vi "Scan Engine EtherCAT Slave.vi"(8 "error in (no error)":errorcluster, 11 "Node Ptr":T1 format="%.0x") -> (0 "error out":errorcluster)   [LabVIEW 2020, in "SEECD System Explorer.lvlib"]
uses:
  SEECD System Explorer.lvlib
  <vilib>/NI VeriStand/Custom Device API/Custom Device API.lvlib
  Shared/Globals/Property Strings.vi
  Shared/SEECD Shared.lvlib
  <vilib>/NI VeriStand/Custom Device API/Set Item Property (U16).vi
  <vilib>/NI VeriStand/Custom Device API/Set Item Property (Boolean).vi
  <vilib>/NI VeriStand/Custom Device API/Custom Device Item Ref.ctl
panel:
  in  "Prepend":bool caption="Prepend slave position to name"
  in  "SHDocVw.IWebBrowser2":refnum<k7>(container)
  in  "Slave Position":u16
  in  "Header":cluster{"Section Name":string}={"Section Name"="NI-914x Chassis"}
  in  "Name":string
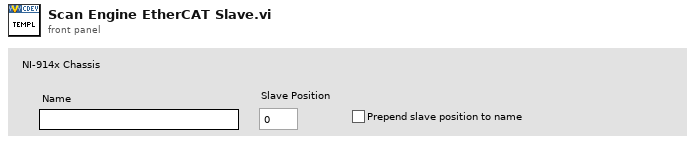
[diagram p1: front panel]
types:
  T1 = typedef "Custom Device API.lvlib/Custom Device Item Ref.ctl" = u64
  T2 = typedef "Custom Device API.lvlib/Custom Device Commands.ctl" = enum16{"Default", "Item renamed", "Shutdown", "Dynamic button pressed"}
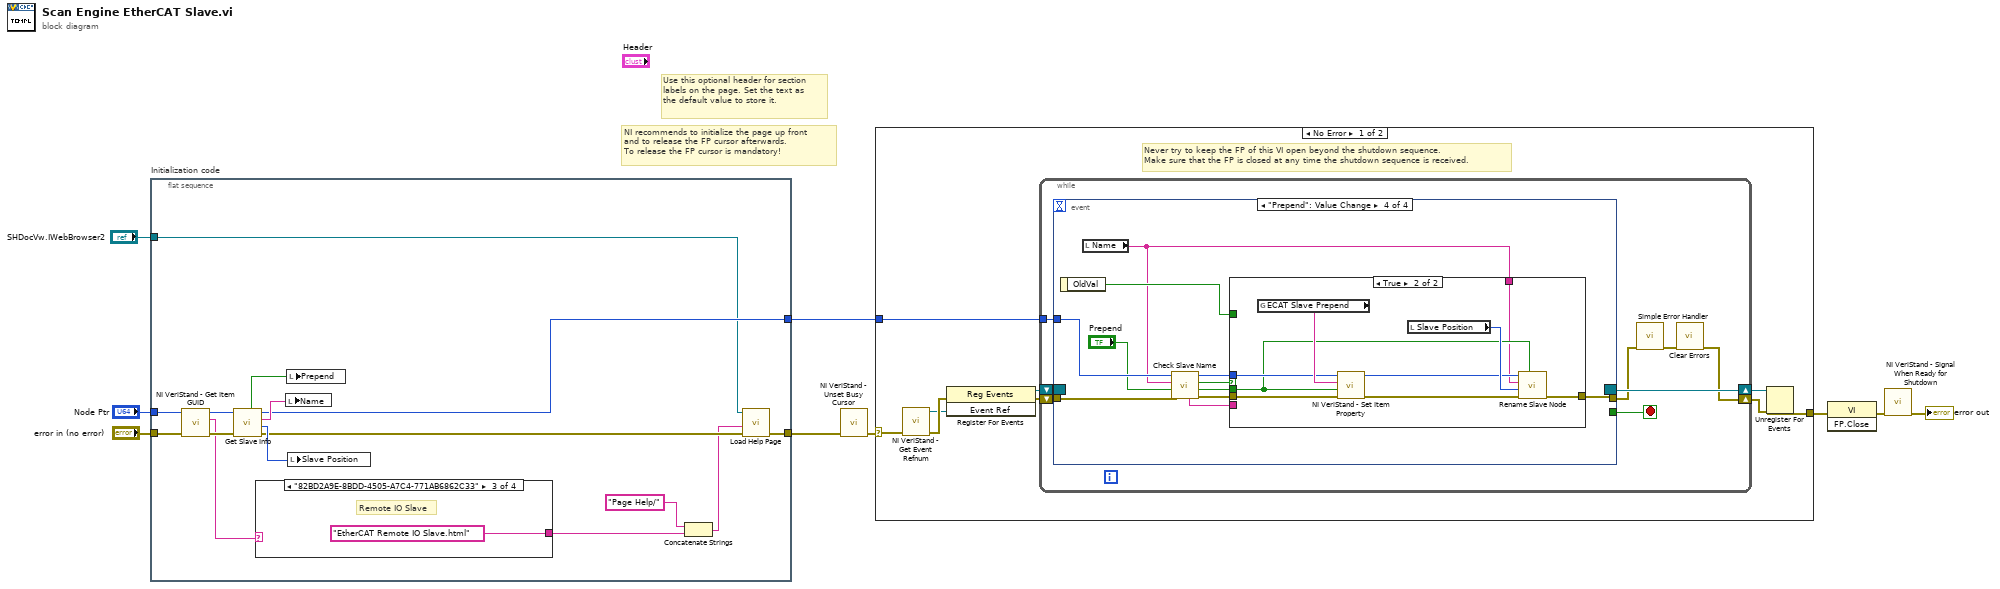
[diagram p0: block diagram]
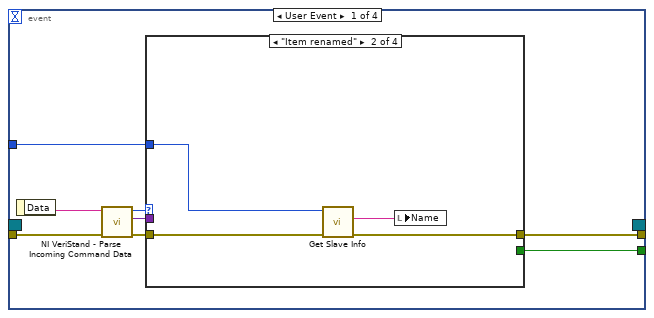
[diagram p2: hidden frame]
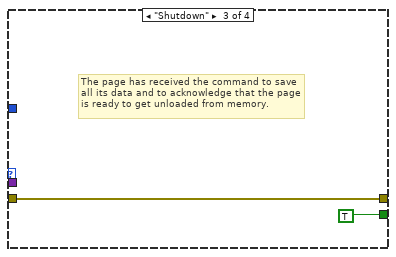
[diagram p4: hidden frame]
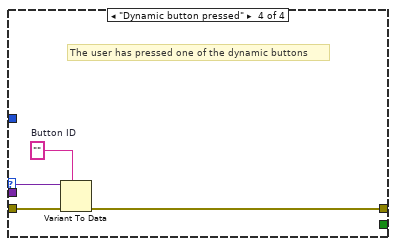
[diagram p5: hidden frame]
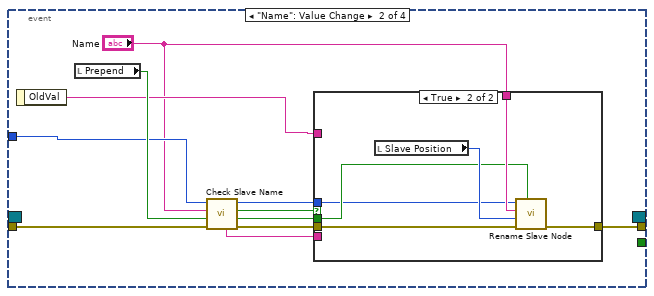
[diagram p6: hidden frame]
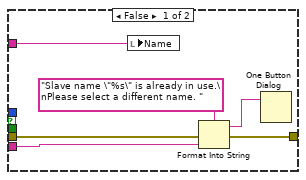
[diagram p7: hidden frame]
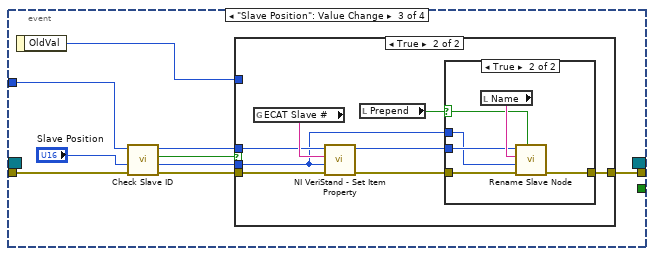
[diagram p8: hidden frame]
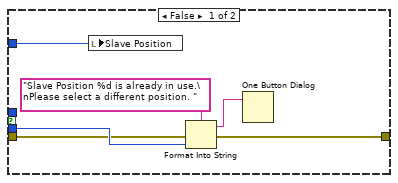
[diagram p9: hidden frame]
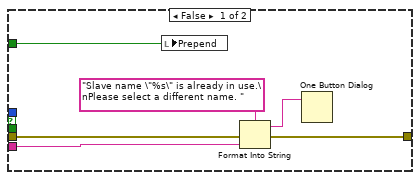
[diagram p11: hidden frame]
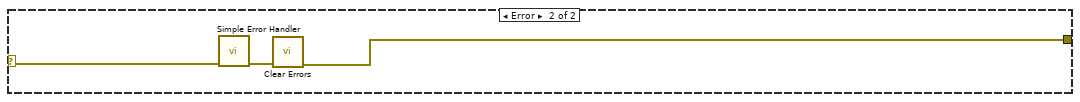
[diagram p12: hidden frame]
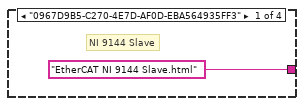
[diagram p13: hidden frame]
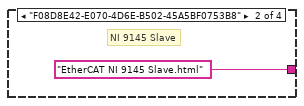
[diagram p14: hidden frame]
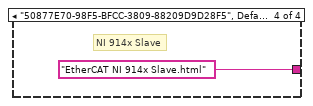
[diagram p15: hidden frame]
diagram:
  # "Use this optional header for section labels on the page. Set the text as the default value to store it."
  # "NI recommends to initialize the page up front\nand to release the FP cursor afterwards.\nTo release the FP cursor is mandatory!"
  n1 = flat-sequence "Initialization code" {
    tunnel: "error in (no error)" -> [w21]
    tunnel: "Node Ptr" -> [w18]
    tunnel: [w22] -> w3
    tunnel: "SHDocVw.IWebBrowser2" -> [w13]
    tunnel: [w15] -> w1
    frame #0 {
      n2 = call <vilib>:"NI VeriStand - Get Item GUID.vi"("error in (no error)"=w21, "Item Ref in"=w18) -> ("error out"=w19:errorcluster, "GUID"=w16:string, "Item Ref out"=w17:T1)  [unwired: 7 in]
      n3 = call "Get Slave Info.vi"("error in (no error)"=w19, "Item Ref in"=w17) -> ("error out"=w14:errorcluster, "Slave #"=w23:u16, "Slave Name"=w24:string, "Item Ref out"=w22:T1, "Prepend"=w20:bool)  [unwired: 4 in, 1 out]
      n4 = case shown="\"82BD2A9E-8BDD-4505-A7C4-771AB6862C33\"" w16 {
        tunnel: ["EtherCAT NI 9144 Slave.html" ("name or relative path") "EtherCAT NI 9145 Slave.html" ("name or relative path") "EtherCAT Remote IO Slave.html" ("name or relative path") "EtherCAT NI 914x Slave.html" ("name or relative path")] -> w12
        frame "0967D9B5-C270-4E7D-AF0D-EBA564935FF3" {
          # "NI 9144 Slave"
        }
        frame "F08D8E42-E070-4D6E-B502-45A5BF0753B8" {
          # "NI 9145 Slave"
        }
        frame "82BD2A9E-8BDD-4505-A7C4-771AB6862C33" {
          # "Remote IO Slave"
        }
        frame "50877E70-98F5-BFCC-3809-88209D9D28F5", Default {
          # "NI 914x Slave"
        }
      }
      n5 = local write "Name"(w24) -> ()
      n6 = local write "Prepend"(w20) -> ()
      n7 = local write "Slave Position"(w23) -> ()
      n8 = Concatenate Strings("Page Help/" ("name or relative path"), w12) -> (w10:string)
      n9 = call "Load Help Page.vi"("error in (no error)"=w14, "HTML File to Load"=w10, "Browser"=w13) -> ("error out"=w15:errorcluster)  [unwired: 8 in]
    }
  }
  n10 = call <vilib>:"NI VeriStand - Unset Busy Cursor.vi"("error in (no error)"=w1) -> ("error out"=w5:errorcluster)  [unwired: 10 out]
  n11 = case shown="No Error" w5 {
    selector: w5 -> [w29 w146]
    tunnel: [w34 w144] -> w9
    tunnel: w3 -> [w30 _]
    frame No Error {
      # "Never try to keep the FP of this VI open beyond the shutdown sequence.\nMake sure that the FP is closed at any time the shutdown sequence is received."
      n12 = call <vilib>:"NI VeriStand - Get Event Refnum.vi"("error in (no error)"=w29) -> ("error out"=w37:errorcluster, "Event Ref"=w33:refnum<user-event>)  [unwired: 9 out]
      n13 = register-events(error in=w37, w33) -> (reference out=w31:refnum<event-registration>, error out=w32:errorcluster)  [unwired: 1 in]
      n14 = while {
        tunnel: w30 -> [w41]
        shift-right: [w38] -> w35
        shift-left: w32 -> [w44]
        shift-right: [w45] -> w36
        shift-left: w31 -> [w43]
        stop <- w42 stop-if-true
        n15 = event shown="[3] \"Prepend\": Value Change" {
          selector: w43 -> [_ _ _ _]
          dyn-events: [_ _ _ _] -> w45
          timeout: _ -> [_ _ _ _]
          tunnel: w44 -> [w53 w70 w92 w122]
          tunnel: [w49 _ _ _] -> w42
          tunnel: [w48 w69 w88 w121] -> w40
          tunnel: w41 -> [w47 w67 w91 w120]
          event User Event {
            n16 = event-data() -> ("Data"=w52:string)  [unwired: 1 out]
            n17 = call <vilib>:"NI VeriStand - Parse Incoming Command Data.vi"("error in (no error)"=w53, "Incoming data"=w52) -> ("error out"=w51:errorcluster, "Outgoing data"=w46:variant, "Action"=w50:T2)  [unwired: 7 out]
            n18 = case shown="\"Item renamed\"" w50 {
              tunnel: w51 -> [w54 w58 w59 w64]
              tunnel: [_ _ TRUE _] -> w49
              tunnel: [w54 w57 w59 w61] -> w48
              tunnel: w47 -> [_ w55 _ _]
              tunnel: w46 -> [_ _ _ w63]
              frame "Default", Default {
              }
              frame "Item renamed" {
                n19 = call "Get Slave Info.vi"("error in (no error)"=w58, "Item Ref in"=w55) -> ("error out"=w57:errorcluster, "Slave Name"=w56:string)  [unwired: 4 in, 4 out]
                n20 = local write "Name"(w56) -> ()
              }
              frame "Shutdown" {
                # "The page has received the command to save all its data and to acknowledge that the page is ready to get unloaded from memory."
              }
              frame "Dynamic button pressed" {
                w62 = ""  # Button ID
                # "The user has pressed one of the dynamic buttons"
                n21 = Variant To Data(error in=w64, type=w62, Variant=w63) -> (error out=w61:errorcluster)  [unwired: 1 out]
              }
            }
          }
          event "Name": Value Change {
            n22 = event-data() -> ("OldVal"=w66:string)  [unwired: 1 out]
            n23 = local read "Prepend"() -> (w68:bool)
            n24 = call "Check Slave Name.vi"("error in (no error)"=w70, "Prepend in"=w68, "Slave Name In"="Name", "Item Ref in"=w67) -> ("error out"=w73:errorcluster, "Prepend out"=w72:bool, "Available?"=w74:bool, "Item Ref out"=w75:T1, "Slave Name"=w71:string)  [unwired: 3 in]
            n25 = case shown="True" w74 {
              tunnel: [w79 w87] -> w69
              tunnel: w73 -> [w80 w84]
              tunnel: w75 -> [_ w82]
              tunnel: w72 -> [_ w83]
              tunnel: w71 -> [w77 _]
              tunnel: "Name" -> [_ w85]
              tunnel: w66 -> [w76 _]
              frame False {
                n26 = local write "Name"(w76) -> ()
                n27 = Format Into String(format string="Slave name \"%s\" is already in use.\nPlease select a different name. ", error in=w80, w77) -> (resulting string=w78:string, error out=w79:errorcluster)  [unwired: 1 in]
                n28 = One Button Dialog(message=w78) -> ()  [unwired: 1 in, 1 out]
              }
              frame True {
                n29 = local read "Slave Position"() -> (w86:u16)
                n30 = call "Rename Slave Node.vi"("Prepend"=w83, "error in (no error)"=w84, "Slave #"=w86, "Slave Name"=w85, "Item Ref in"=w82) -> ("error out"=w87:errorcluster)  [unwired: 5 in, 1 out]
              }
            }
          }
          event "Slave Position": Value Change {
            n31 = event-data() -> ("OldVal"=w90:u16)  [unwired: 1 out]
            n32 = call "Check Slave ID.vi"("error in (no error)"=w92, "Slave ID in"="Slave Position", "Item Ref in"=w91) -> ("error out"=w96:errorcluster, "Slave ID out"=w94:u16, "Available?"=w95:bool, "Item Ref out"=w93:T1)  [unwired: 5 in]
            n33 = case shown="True" w95 {
              tunnel: [w98 w110] -> w88
              tunnel: w96 -> [w99 w108]
              tunnel: w93 -> [_ w106]
              tunnel: w94 -> [w101 w104]
              tunnel: w90 -> [w97 _]
              frame False {
                n34 = local write "Slave Position"(w97) -> ()
                n35 = Format Into String(format string="Slave Position %d is already in use.\nPlease select a different position. ", error in=w99, w101) -> (resulting string=w100:string, error out=w98:errorcluster)  [unwired: 1 in]
                n36 = One Button Dialog(message=w100) -> ()  [unwired: 1 in, 1 out]
              }
              frame True {
                n37 = global read "Property Strings.vi" "ECAT Slave #"() -> (w109:string)
                n38 = call-poly <vilib>:"NI VeriStand - Set Item Property.vi"("error in (no error)"=w108, "Value"=w104, "Property Name"=w109, "Item Ref in"=w106) -> ("error out"=w107:errorcluster, "Item Ref out"=w105:T1)  [unwired: 5 in, 1 out]
                n39 = local read "Prepend"() -> (w103:bool)
                n40 = case shown="True" w103 {
                  selector: w103 -> [_ w112]
                  tunnel: [w111 w117] -> w110
                  tunnel: w107 -> [w111 w115]
                  tunnel: w105 -> [_ w114]
                  tunnel: w104 -> [_ w113]
                  frame False {
                  }
                  frame True {
                    n41 = local read "Name"() -> (w116:string)
                    n42 = call "Rename Slave Node.vi"("Prepend"=w112, "error in (no error)"=w115, "Slave #"=w113, "Slave Name"=w116, "Item Ref in"=w114) -> ("error out"=w117:errorcluster)  [unwired: 5 in, 1 out]
                  }
                }
              }
            }
          }
          event "Prepend": Value Change {
            n43 = event-data() -> ("OldVal"=w123:bool)  [unwired: 1 out]
            n44 = local read "Name"() -> (w119:string)
            n45 = call "Check Slave Name.vi"("error in (no error)"=w122, "Prepend in"="Prepend", "Slave Name In"=w119, "Item Ref in"=w120) -> ("error out"=w126:errorcluster, "Prepend out"=w125:bool, "Available?"=w127:bool, "Item Ref out"=w128:T1, "Slave Name"=w124:string)  [unwired: 3 in]
            n46 = case shown="True" w127 {
              tunnel: [w131 w143] -> w121
              tunnel: w126 -> [w132 w140]
              tunnel: w128 -> [_ w138]
              tunnel: w125 -> [_ w136]
              tunnel: w123 -> [w134 _]
              tunnel: w124 -> [w129 _]
              tunnel: w119 -> [_ w135]
              frame False {
                n47 = local write "Prepend"(w134) -> ()
                n48 = Format Into String(format string="Slave name \"%s\" is already in use.\nPlease select a different name. ", error in=w132, w129) -> (resulting string=w130:string, error out=w131:errorcluster)  [unwired: 1 in]
                n49 = One Button Dialog(message=w130) -> ()  [unwired: 1 in, 1 out]
              }
              frame True {
                n50 = global read "Property Strings.vi" "ECAT Slave Prepend"() -> (w141:string)
                n51 = call-poly <vilib>:"NI VeriStand - Set Item Property.vi"("error in (no error)"=w140, "Value"=w136, "Property Name"=w141, "Item Ref in"=w138) -> ("error out"=w139:errorcluster, "Item Ref out"=w137:T1)  [unwired: 5 in, 1 out]
                n52 = local read "Slave Position"() -> (w142:u16)
                n53 = call "Rename Slave Node.vi"("Prepend"=w136, "error in (no error)"=w139, "Slave #"=w142, "Slave Name"=w135, "Item Ref in"=w137) -> ("error out"=w143:errorcluster)  [unwired: 5 in, 1 out]
              }
            }
          }
        }
        n54 = call <vilib>:"Simple Error Handler.vi"("error in (no error)"=w40) -> ("error out"=w39:errorcluster)  [unwired: 1 in, 7 out]
        n55 = call <vilib>:"Clear Errors.vi"("error in (no error)"=w39) -> ("error out"=w38:errorcluster)  [unwired: 1 in, 5 out]
      }
      n56 = Unregister For Events(event registration refnum=w36, error in=w35) -> (error out=w34:errorcluster)
    }
    frame Error {
      n57 = call <vilib>:"Simple Error Handler.vi"("error in (no error)"=w146) -> ("error out"=w145:errorcluster)  [unwired: 1 in, 7 out]
      n58 = call <vilib>:"Clear Errors.vi"("error in (no error)"=w145) -> ("error out"=w144:errorcluster)  [unwired: 1 in, 5 out]
    }
  }
  n59 = invoke class="VI" method="FP.Close"(error in=w9) -> (error out=w8:errorcluster)  [unwired: 2 in, 2 out]
  n60 = call <vilib>:"NI VeriStand - Signal When Ready for Shutdown.vi"("error in (no error)"=w8) -> ("error out"=→"error out":errorcluster)  [unwired: 10 out]
